vi "LoadDatabaseList.vi"(8 "error in":errorcluster) -> (0 "error out":errorcluster, 2 "filenames":string[](array[string]), 3 "path out":path)   [LabVIEW 2013]
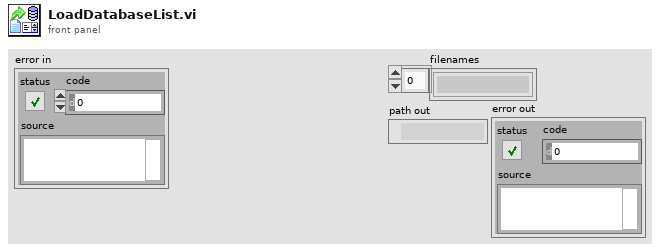
[diagram p1: front panel]
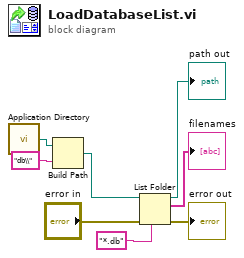
[diagram p0: block diagram]
diagram:
  n1 = call <vilib>:"Application Directory.vi"() -> ("Application Directory"=w5:path)
  n2 = Build Path(base path=w5, name or relative path="db\\") -> (appended path=w7:path)
  n3 = List Folder(path=w7, pattern="*.db", error in="error in") -> (path out=→"path out":path, filenames=→"filenames":string[], error out=→"error out":errorcluster)  [unwired: 1 in, 1 out]
